vi "Rank.vi"(10 "tol":dbl, 11 "R":T1) -> (3 "Numeric":i16)   [LabVIEW 2014]
uses:
  <vilib>/Analysis/Matrix/Datatypes/RealMatrix.ctl
  <vilib>/Analysis/Matrix/NI_Matrix.lvlib
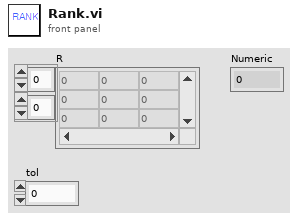
[diagram p1: front panel]
types:
  T1 = typedef "NI_Matrix.lvlib/RealMatrix.ctl" = dbl[][]
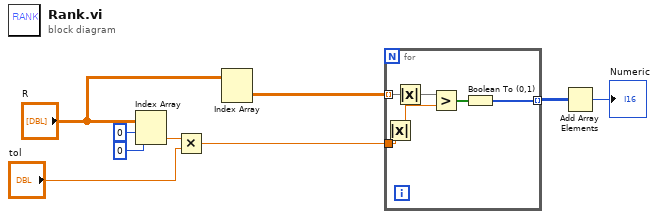
[diagram p0: block diagram]
diagram:
  n1 = Index Array(array="R", index (row)=0, index (col)=0 ("disabled index (col)")) -> (element=w3:dbl)
  n2 = Multiply(x=w3, y="tol") -> (x*y=w7:dbl)
  n3 = Index Array(array="R") -> (element=w6:T1)  [unwired: 2 in]
  n4 = for {
    tunnel: w6 -> [w15] mode=indexing
    tunnel: w7 -> [w14]
    tunnel: [w12] -> w8 mode=indexing
    n5 = Absolute Value(x=w14) -> (abs(x)=w11:dbl)
    n6 = Absolute Value(x=w15) -> (abs(x)=w10:dbl[])
    n7 = Greater?(x=w10, y=w11) -> (0:w13:bool[])
    n8 = Boolean To (0,1)(Boolean=w13) -> (0, 1=w12:i16[])
  }
  n9 = Add Array Elements(numeric array=w8) -> (sum=→"Numeric":i16)
